vi "GetElapsedMinsSecs.vi"(8 "error in (no error)":errorcluster, 11 "Op Start Time":timestamp) -> (0 "error out":errorcluster, 1 "Elapsed mm:ss":string, 2 "ElapsedTime":string, 3 "Elapsed secs since start":i32)   [LabVIEW 2024]
panel:
  in  "Function":T1(ring)=enum."Get elapsed time (msec)"
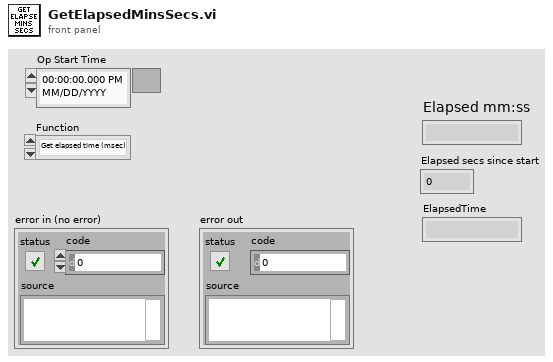
[diagram p1: front panel]
types:
  T1 = enum16{"Init timer", "Get elapsed time (msec)", "Stop timer"}
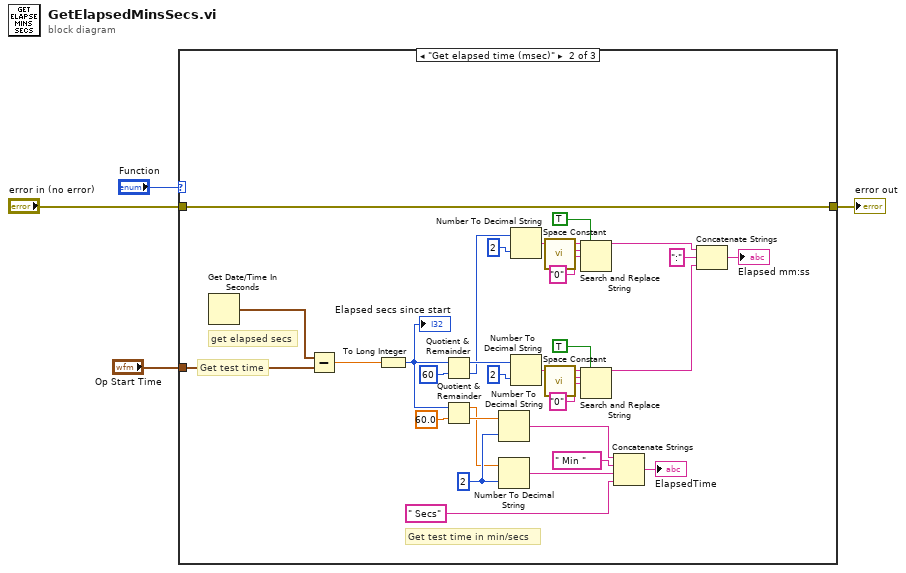
[diagram p0: block diagram]
diagram:
  n1 = case shown="\"Get elapsed time (msec)\"" "Function" {
    tunnel: [w5 w36 w37] -> w3
    tunnel: "error in (no error)" -> [w5 w36 w37]
    tunnel: "Op Start Time" -> [_ w24 _]
    frame "Init timer", Default {
    }
    frame "Get elapsed time (msec)" {
      w31 = i16 2 ("width (-)")
      # "Get test time"
      # "Get test time in min/secs"
      # "get elapsed secs"
      n2 = Get Date/Time In Seconds() -> (seconds since 1Jan1904=w34:timestamp)
      n3 = Subtract(x=w34, y=w24) -> (x-y=w33:dbl)
      n4 = To Long Integer(number=w33) -> (32bit integer=w35:i32)
      "Elapsed secs since start" <- w35
      n5 = Quotient & Remainder(x=w35, y=60) -> (x-y*floor(x/y)=w15:i32, floor(x/y)=w14:i32)
      n6 = Quotient & Remainder(x=w35, y=60.0) -> (x-y*floor(x/y)=w29:dbl, floor(x/y)=w30:dbl)
      n7 = Number To Decimal String(number=w30, width (-)=w31) -> (decimal integer string=w25:string)
      n8 = Number To Decimal String(number=w29, width (-)=w31) -> (decimal integer string=w27:string)
      n9 = Number To Decimal String(number=w14, width (-)=i16 2) -> (decimal integer string=w17:string)
      n10 = Number To Decimal String(number=w15, width (-)=i16 2) -> (decimal integer string=w21:string)
      n11 = call <vilib>:"Space Constant.vi"() -> ("String"=w18:string)
      n12 = call <vilib>:"Space Constant.vi"() -> ("String"=w20:string)
      n13 = Search and Replace String(replace all?=TRUE ("replace all? (F)"), input string=w17, search string=w18, replace string="0" ("replace string (\"\")")) -> (result string=w19:string)  [unwired: 4 in, 3 out]
      n14 = Search and Replace String(replace all?=TRUE ("replace all? (F)"), input string=w21, search string=w20, replace string="0" ("replace string (\"\")")) -> (result string=w22:string)  [unwired: 4 in, 3 out]
      n15 = Concatenate Strings(w25, " Min " ("string"), w27, " Secs" ("string")) -> (→"ElapsedTime":string)
      n16 = Concatenate Strings(w19, ":" ("string"), w22) -> (→"Elapsed mm:ss":string)
    }
    frame "Stop timer" {
    }
  }
  "error out" <- w3
